vi "ELVIS III v1.0 Configure DI Mode.vi"(7 "Apply Bitmask?":bool=TRUE, 8 "error in (no error)":errorcluster, 10 "Bitmask Array":bool[][](array[boolean]), 11 "myRIO FPGA Ref In":T1) -> (0 "error out":errorcluster)   [LabVIEW 2021]
uses:
  <vilib>/myRIO/Common/Instrument Driver Framework/Utilities/typedefs/Generic FPGA Reference.ctl
  <vilib>/myRIO/Common/Instrument Driver Framework/ELVIS III v1.0/DO Block/typedefs/ELVIS III DO Block FPGA Reference.ctl
  <vilib>/myRIO/Common/Instrument Driver Framework/ELVIS III v1.0/Resource Manager/typedefs/ELVIS III v1.0 Connector List.ctl
  <vilib>/Utility/error.llb/Error Cluster From Error Code.vi
  <vilib>/rvi/errors/niLvFpgaAdjustHostInterfaceError.vi
  <vilib>/rvi/interface/nirviReadWriteControl/nirviReadWriteControl.xnode
  NiFpgaLv.dll
  <vilib>/rvi/interface/Simulation/niFpgaSimulationCallBeginRW.vi
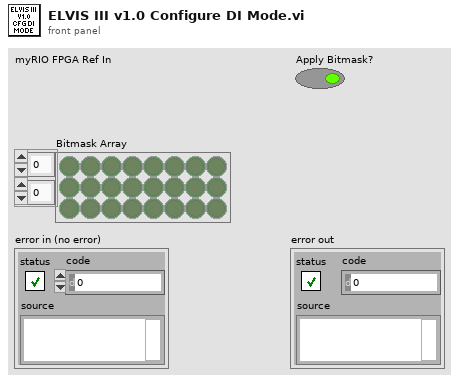
[diagram p1: front panel]
types:
  T1 = typedef "Generic FPGA Reference.ctl" = refnum<k20>
  T2 = typedef "ELVIS III DO Block FPGA Reference.ctl" = refnum<k20>
  T3 = typedef "ELVIS III v1.0 Connector List.ctl" = enum32{"None", "ConnectorA", "ConnectorB"}
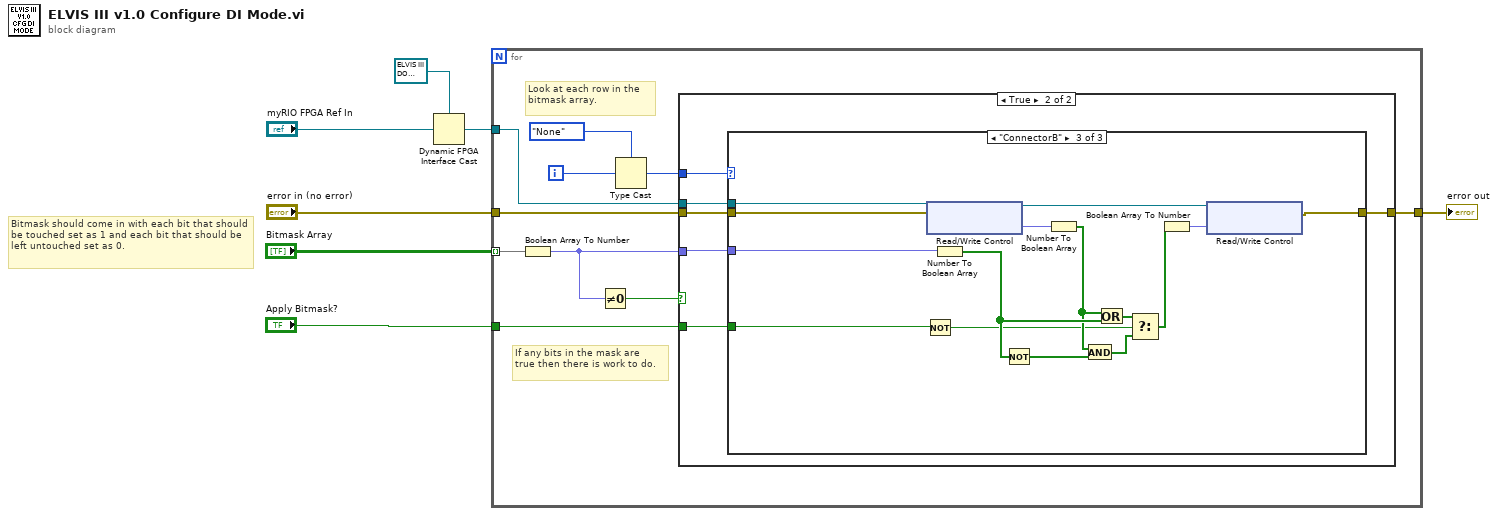
[diagram p0: block diagram]
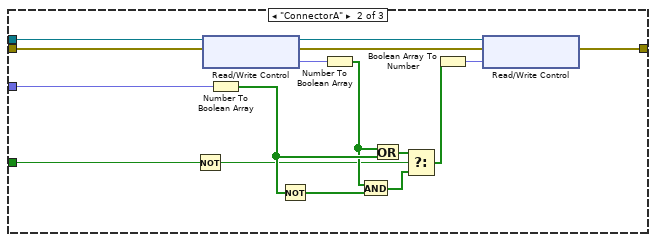
[diagram p4: hidden frame]
diagram:
  # "Bitmask should come in with each bit that should be touched set as 1 and each bit that should be left untouched set as 0."
  n1 = Dynamic FPGA Interface Cast(Session In=T2 refnum ("FPGA Interface"), Type="myRIO FPGA Ref In") -> (Session Out=w4:T2)
  n2 = for {
    tunnel: w4 -> [w17]
    tunnel: "error in (no error)" -> [w16]
    tunnel: [w15] -> w6
    tunnel: "Bitmask Array" -> [w11] mode=indexing
    tunnel: "Apply Bitmask?" -> [w8]
    i -> [w14]
    # "If any bits in the mask are\ntrue then there is work to do."
    # "Look at each row in the bitmask array."
    n3 = Boolean Array To Number(Boolean array=w11) -> (number=w10:fxp<+,20,20>)
    n4 = Not Equal To 0?(x=w10) -> (x != 0?=w9:bool)
    n5 = Type Cast(type=ELVIS_III_v1.0_Connector_List."None" ("Connector List"), x=w14) -> (*(type *) &x=w13:T3)
    n6 = case shown="True" w9 {
      tunnel: w17 -> [_ w24]
      tunnel: w16 -> [w18 w23]
      tunnel: [w18 w22] -> w15
      tunnel: w13 -> [_ w21]
      tunnel: w10 -> [_ w20]
      tunnel: w8 -> [_ w19]
      frame False {
        # "There are no bits to change for this connector."
      }
      frame True {
        n7 = case shown="\"ConnectorB\"" w21 {
          tunnel: w24 -> [_ w37 w56]
          tunnel: w23 -> [w25 w38 w55]
          tunnel: [w25 w41 w54] -> w22
          tunnel: w20 -> [_ w39 w53]
          tunnel: w19 -> [_ w40 w52]
          frame "None", Default {
            # "Do Nothing"
          }
          frame "ConnectorA" {
            n8 = Not(x=w40) -> (.not. x?=w26:bool)
            n9 = xnode "Read/Write Control"("FPGA VI Reference In"=w37, "error in"=w38) -> ("FPGA VI Reference Out"=w31:T2, "error out"=w29:errorcluster, "DIO.A_19:0.DIR"=w32:fxp<+,20,20>)
            n10 = Number To Boolean Array(number=w39) -> (Boolean array=w35:bool[])
            n11 = Not(x=w35) -> (.not. x?=w34:bool[])
            n12 = Number To Boolean Array(number=w32) -> (Boolean array=w27:bool[])
            n13 = And(x=w27, y=w34) -> (x .and. y?=w33:bool[])
            n14 = Or(x=w27, y=w35) -> (x .or. y?=w36:bool[])
            n15 = Select(t=w36, s=w26, f=w33) -> (s? t:f=w28:bool[])
            n16 = Boolean Array To Number(Boolean array=w28) -> (number=w30:fxp<+,20,20>)
            n17 = xnode "Read/Write Control"("FPGA VI Reference In"=w31, "error in"=w29, "DIO.A_19:0.DIR"=w30) -> ("error out"=w41:errorcluster)  [unwired: 1 out]
          }
          frame "ConnectorB" {
            n18 = Not(x=w52) -> (.not. x?=w42:bool)
            n19 = xnode "Read/Write Control"("FPGA VI Reference In"=w56, "error in"=w55) -> ("FPGA VI Reference Out"=w46:T2, "DIO.B_19:0.DIR"=w47:fxp<+,20,20>)  [unwired: 1 out]
            n20 = Number To Boolean Array(number=w53) -> (Boolean array=w50:bool[])
            n21 = Not(x=w50) -> (.not. x?=w49:bool[])
            n22 = Number To Boolean Array(number=w47) -> (Boolean array=w43:bool[])
            n23 = And(x=w43, y=w49) -> (x .and. y?=w48:bool[])
            n24 = Or(x=w43, y=w50) -> (x .or. y?=w51:bool[])
            n25 = Select(t=w51, s=w42, f=w48) -> (s? t:f=w44:bool[])
            n26 = Boolean Array To Number(Boolean array=w44) -> (number=w45:fxp<+,20,20>)
            n27 = xnode "Read/Write Control"("FPGA VI Reference In"=w46, "DIO.B_19:0.DIR"=w45) -> ("error out"=w54:errorcluster)  [unwired: 1 in, 1 out]
          }
        }
      }
    }
  }
  "error out" <- w6
